vi "Test XY Graph to ITX Graph.vi"() -> ()   [LabVIEW 2019]
uses:
  LV-Data.ITX/LV-Data.ITX.lvclass
panel:
  out "file":path=path "C:/Users/voodoo.SEAGATE/Desktop/datatest/datatest.000019.itx"
  out "XY Graph":cluster{i32[], dbl[]}[](graph)
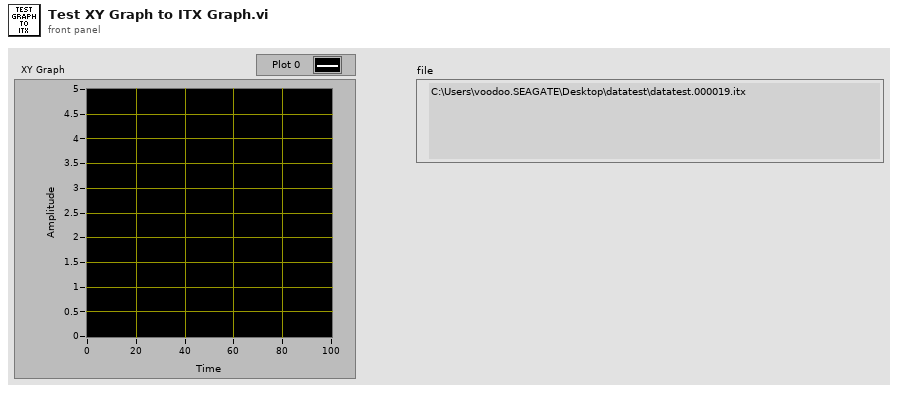
[diagram p1: front panel]
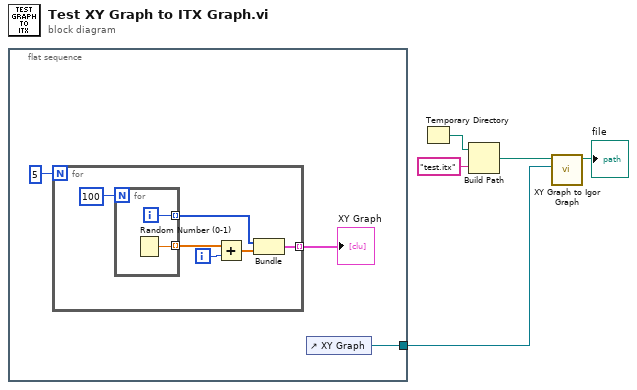
[diagram p0: block diagram]
diagram:
  n1 = flat-sequence {
    tunnel: [w6] -> w1
    frame #0 {
      n2 = for {
        N: 5 -> [_]
        tunnel: [w9] -> w8 mode=indexing
        i -> [w12]
        n3 = for {
          N: 100 -> [_]
          tunnel: [w16] -> w13 mode=indexing
          tunnel: [w15] -> w11 mode=indexing
          i -> [w15]
          n4 = Random Number (0-1)() -> (number: 0 to 1=w16:dbl)
        }
        n5 = Add(x=w13, y=w12) -> (x+y=w10:dbl[])
        n6 = Bundle(w11, w10) -> (w9:cluster{i32[], dbl[]})  [unwired: 1 in]
      }
      "XY Graph" <- w8
      n7 = control-ref of="XY Graph"() -> (w6:refnum<vi>)
    }
  }
  n8 = Temporary Directory() -> (w2:path)
  n9 = Build Path(base path=w2, name or relative path="test.itx") -> (appended path=w4:path)
  n10 = call "XY Graph to Igor Graph.vi"("XY Graph Reference"=w1, "Path"=w4) -> ("file"=→"file":path)  [unwired: 8 in, 1 out]
